vi "Send Status String.vi"(8 "error in (no error)":errorcluster, 10 "String":string, 11 "Message Enqueuer in":refnum<class "Message Enqueuer.lvclass">) -> (0 "error out":errorcluster, 3 "Message Enqueuer out":refnum<class "Message Enqueuer.lvclass">)   [LabVIEW 2016, in "Generic UI Actor.lvlib" / "Update Status Display.lvclass"]
uses:
  <userlib>/Common Components/User Interface/Messages/Update Status Display/Update Status Display.lvclass
  <vilib>/ActorFramework/Message Enqueuer/Message Enqueuer.lvclass
  C:/Program Files (x86)/National Instruments/LabVIEW 2016/vi.lib/ActorFramework/Message/Message.lvclass
  <vilib>/ActorFramework/Message Enqueuer/Message Enqueuer.lvclass/Message Enqueuer.ctl
  <vilib>/ActorFramework/Message Priority Queue/Priority Enqueue.vi
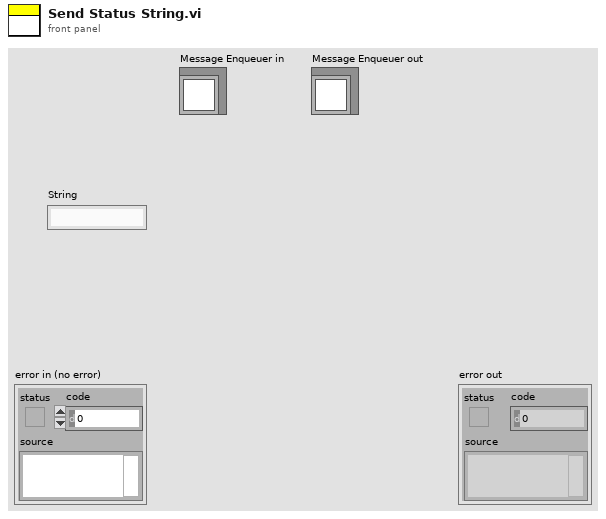
[diagram p1: front panel]
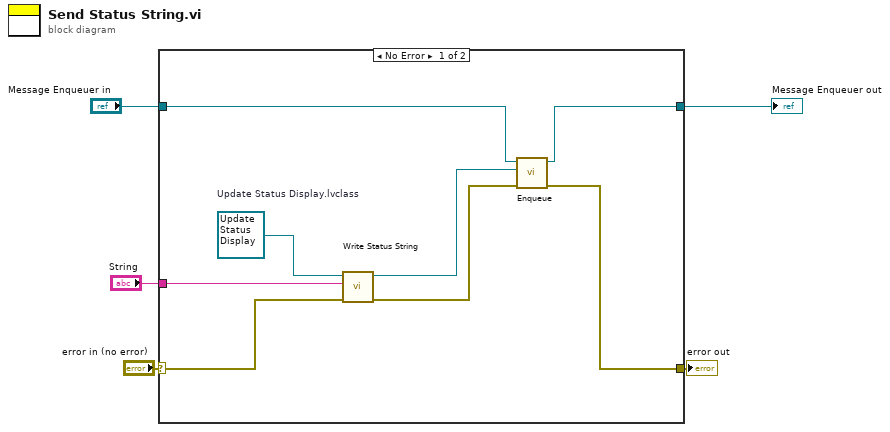
[diagram p0: block diagram]
diagram:
  n1 = case shown="No Error" "error in (no error)" {
    selector: "error in (no error)" -> [w11 w15]
    tunnel: [w8 w15] -> w4
    tunnel: "String" -> [w12 _]
    tunnel: "Message Enqueuer in" -> [w7 w14]
    tunnel: [w6 w14] -> w1
    frame No Error {
      w13 = refnum<class "Update Status Display.lvclass"> refnum  # Update Status Display.lvclass
      n2 = call <userlib>:"Write Status String.vi"("error in (no error)"=w11, "Status String"=w12, "Update Status Display in"=w13) -> ("error out"=w9:errorcluster, "Update Status Display out"=w10:refnum<class "Update Status Display.lvclass">)  [unwired: 7 in]
      n3 = call <vilib>:"Enqueue.vi"("error in (no error)"=w9, "Message"=w10, "Message Enqueuer in"=w7) -> ("error out"=w8:errorcluster, "Message Enqueuer out"=w6:refnum<class "Message Enqueuer.lvclass">)  [unwired: 7 in]
    }
    frame Error {
    }
  }
  "error out" <- w4
  "Message Enqueuer out" <- w1
